vi "myRIO_BRig_RT_dataAnalog_enterData__PortA.vi"(4 "input_iState":T1, 5 "input_AI0":u16, 6 "input_iEvent":u16, 7 "input_AI1":u16, 8 "input_iTrial":u16, 9 "input_iBlock":u16, 10 "input_index":i32, 11 "input_dataAnalog":u16[][](array[numeric])) -> (3 "output_dataAnalog":u16[][](array[numeric]))   [LabVIEW 2014]
uses:
  myRIO_BRig_RT__Case_Exp_stateList.ctl
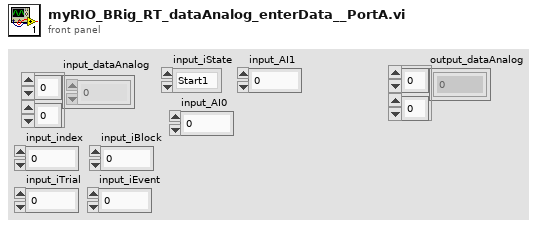
[diagram p1: front panel]
types:
  T1 = typedef "myRIO_BRig_RT__Case_Exp_stateList.ctl" = enum16{"Start1", "Start2", "Start3", "saveSettings1", "saveSettings2", "saveSettings3", "saveSettings4", "saveSettings_LC_ENL_l1", "saveSettings_LC_ENL_l2", "saveSettings_LC_Cue_l1", "saveSettings_LC_Cue_l2", "saveSettings6_LC_l1_Other", "SaveSettings6_LC_l2_Other", "setSettings_Audio", "setSettings_Laser", "initBlock_pre", "initBlock", "initBlock2", "initBlock_post", "initTrial_pre", "initTrial", "initTrial2", "initTrial3", "initTrial4", "initTrial_LC_ENL1", "initTrial_LC_Cue1", "initTrial_LC_Cue1_2", "initTrial_LC_Sel", "initTrial_post", "ENL1_pre", "ENL1", "ENL1_post", "ENL1Penalty_pre", "ENL1Penalty", "ENL2_pre", "ENL2", "ENL2Penalty_pre", "ENL2Penalty", "Cue1_pre", "Cue1", "Cue1_post", "Cue1Penalty_pre", "Cue1Penalty", "Cue2_pre", "Cue2", "Cue2Penalty_pre", "Cue2Penalty", "Selection_pre", "Selection", "Select_post", "SelectReward_pre", "SelectReward", "SelectRewardPost_pre", "SelectRewardPost", "SelectWrong_pre", "SelectWrong", "SelectWrong_post", "SelectTimeout_pre", "SelectTimeout", "SelectTimeout_post", "endTrial_pre", "endTrial1", "endTrial2", "endTrial3", "endTrial_post", "endBlock_pre", "endBlock", "endBlock_post", "endExp", "commConnect", "commUpload_pre", "commUpload_dataBlock", "commUpload_dataCurrent", "commUpload_dataExp", "commUpload_dataLC", "commUpload_dataTrial", "commUpload_post", "saveData_pre", "saveData_dataBlock", "saveData_dataCurrent", "saveData_dataExp", "saveData_dataLC", "saveData_dataTrial", "saveData_post", "empty_endBlock1", "empty_endBlock2", "empty_endTrial1", "empty_endTrial2", "empty_endTrial3", "empty_endTrial4", "empty_endTrial5", "dummyState", "dummyState_endBlock"}
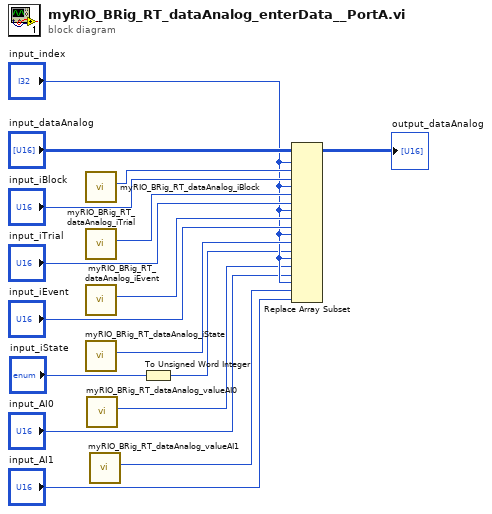
[diagram p0: block diagram]
diagram:
  n1 = call "myRIO_BRig_RT_dataAnalog_iBlock.vi"() -> ("output_iBlock"=w15:i32)  [unwired: 11 in]
  n2 = call "myRIO_BRig_RT_dataAnalog_iTrial.vi"() -> ("output_iTrial"=w13:i32)  [unwired: 11 in]
  n3 = call "myRIO_BRig_RT_dataAnalog_iEvent.vi"() -> ("output_iEvent"=w11:i32)  [unwired: 11 in]
  n4 = call "myRIO_BRig_RT_dataAnalog_iState.vi"() -> ("output_iState"=w9:i32)  [unwired: 11 in]
  n5 = call "myRIO_BRig_RT_dataAnalog_valueAI0.vi"() -> ("output_valueAI0"=w7:i32)  [unwired: 11 in]
  n6 = call "myRIO_BRig_RT_dataAnalog_valueAI1.vi"() -> ("output_valueAI1"=w5:i32)  [unwired: 11 in]
  n7 = To Unsigned Word Integer(number="input_iState") -> (unsigned 16bit integer=w1:u16)
  n8 = Replace Array Subset(array="input_dataAnalog", new element #1="input_iBlock", index (row) #1="input_index", index (col) #1=w15, new element #2="input_iTrial", index (row) #2="input_index", index (col) #2=w13, new element #3="input_iEvent", index (row) #3="input_index", index (col) #3=w11, new element #4=w1, index (row) #4="input_index", index (col) #4=w9, new element #5="input_AI0", index (row) #5="input_index", index (col) #5=w7, new element #6="input_AI1", index (row) #6="input_index", index (col) #6=w5) -> (→"output_dataAnalog":u16[][])
